vi "Cluster_Disable Unlabeled Items.vi"(11 "Cluster Items":T1[](array[typedef])) -> (3 "Cluster Items Out":T1[](array[typedef]))   [LabVIEW 2023]
doc: "Disable cluster items that have no label or where any ancestor item has no label. These cannot be set programatically in an un/bundle by name node."
uses:
  Cluster Element Description.ctl
  <userlib>/_OpenG.lib/array/array.llb/openg_array.lvlib
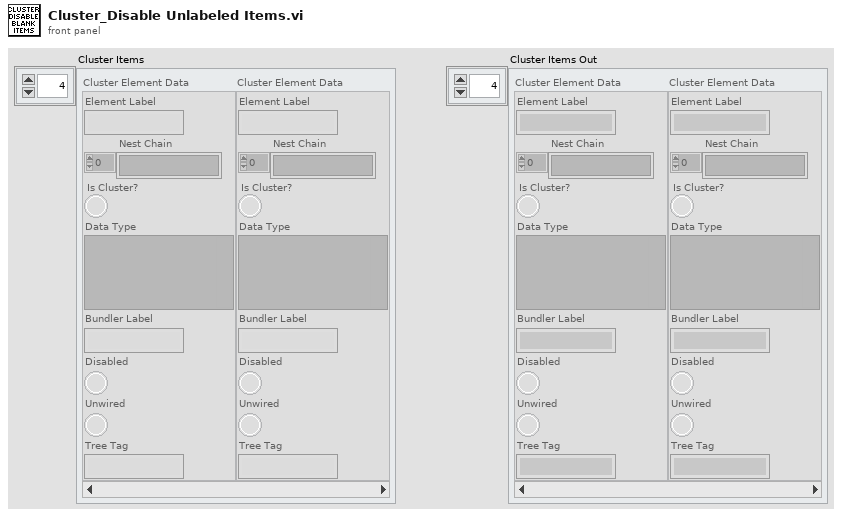
[diagram p1: front panel]
types:
  T1 = typedef "Cluster Element Description.ctl" = cluster{"Element Label":string, "Nest Chain":string[], "Is Cluster?":bool, "Data Type":variant, "Bundler Label":string, "Disabled":bool, "Unwired":bool, "Tree Tag":string}
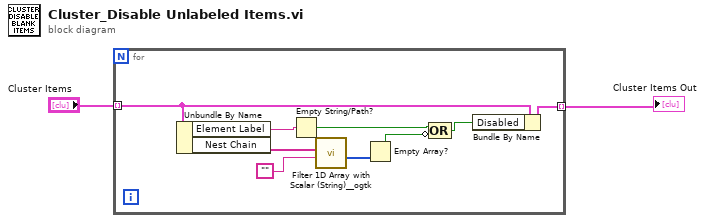
[diagram p0: block diagram]
diagram:
  n1 = for {
    tunnel: "Cluster Items" -> [w7] mode=indexing
    tunnel: [w8] -> w1 mode=indexing
    n2 = Unbundle By Name(w7) -> ("Element Label"=w11:string, "Nest Chain"=w10:string[])
    n3 = Empty String/Path?(string/path=w11) -> (empty?=w6:bool)
    n4 = call <userlib>:"Filter 1D Array with Scalar (String)__ogtk.vi"("items to filter"="", "array"=w10) -> ("filtered item indices"=w3:i32[])  [unwired: 4 in, 1 out]
    n5 = Empty Array?(array=w3) -> (empty?=w5:bool)
    n6 = Compound Arithmetic op=OR(w6, invert w5) -> (w4:bool)
    n7 = Bundle By Name(cluster=w7, "Disabled"=w4) -> (w8:T1)
  }
  "Cluster Items Out" <- w1
